vi "故障码字段定义.vi"(9 "首次调用？":bool, 10 "id":u16, 11 "故障代码":u16) -> (3 "data":T1)   [LabVIEW 2016, in "斯坦道氨氮V2.lvlib"]
uses:
  Alarm interface/Alarm interface.lvlib
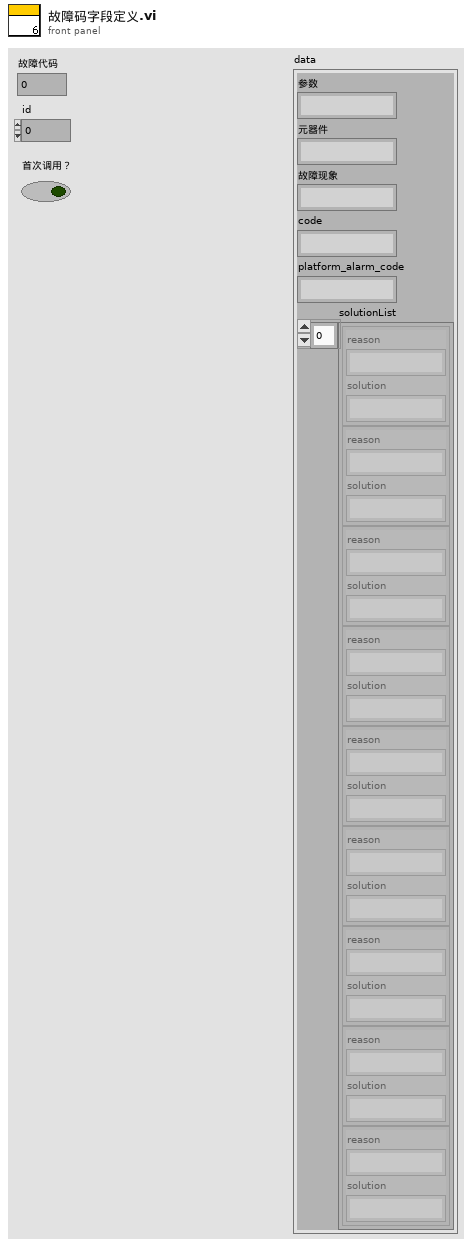
[diagram p1: front panel]
types:
  T1 = typedef "Alarm interface.lvlib/报警短信语音交互.ctl" = cluster{"参数":string, "元器件":string, "故障现象":string, "code":string, "platform_alarm_code":string, "solutionList":cluster{"reason":string, "solution":string}[]}
  T2 = cluster{"table输出":string, "equipVersion":string, string}
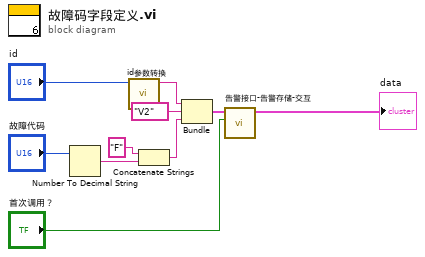
[diagram p0: block diagram]
diagram:
  n1 = Number To Decimal String(number="故障代码") -> (decimal integer string=w3:string)  [unwired: 1 in]
  n2 = call "id参数转换.vi"("id"="id") -> ("table输出"=w10:string)  [unwired: 9 in, 1 out]
  n3 = Concatenate Strings("F" ("字符串"), w3) -> (w1:string)
  n4 = Bundle("table输出"=w10, "equipVersion"="V2", w1) -> (w7:T2)  [unwired: 1 in]
  n5 = call "告警接口-告警存储-交互.vi"("首次调用？"="首次调用？", "筛选输入"=w7) -> ("data"=→"data":T1)  [unwired: 9 in]
